vi "AddPotentialSweep.vi"(0 "deviceName":string, 1 "channel":u8, 2 "repeats":u16=1, 3 "quietTime":sgl, 4 "quietTimeSamplingInterval":sgl=1.0, 5 "startingPot":sgl, 6 "isStartVoltageVsOCP":bool, 7 "error in (no error)":errorcluster, 8 "endingPot":sgl, 9 "isEndVoltageVsOCP":bool, 10 "scanRate":sgl, 11 "samplingInterval":sgl, 12 "approxMaxCurrent":sgl=inf, 13 "isAutoRange":bool=TRUE, 14 "maxAbsoluteCurrent":sgl=inf, 15 "minAbsoluteCurrent":sgl, 16 "alphaFactor":sgl=75.0) -> (27 "error out":errorcluster)   [LabVIEW 2018]
doc: "EXPORT void AisAddPotentialSweep(const char* deviceName, uint8_t channel, uint16_t repeats, float quietTime, float quietTimeSamplingInterval, float startingPot, bool isStartVoltageVsOCP, float endingPot, bool isEndVoltageVsOCP, float scanRate, float samplingInterval, float approxMaxCurrent, bool isAutoRange, float maxAbsoluteCurrent, float minAbsoluteCurrent, float alphaFactor);"
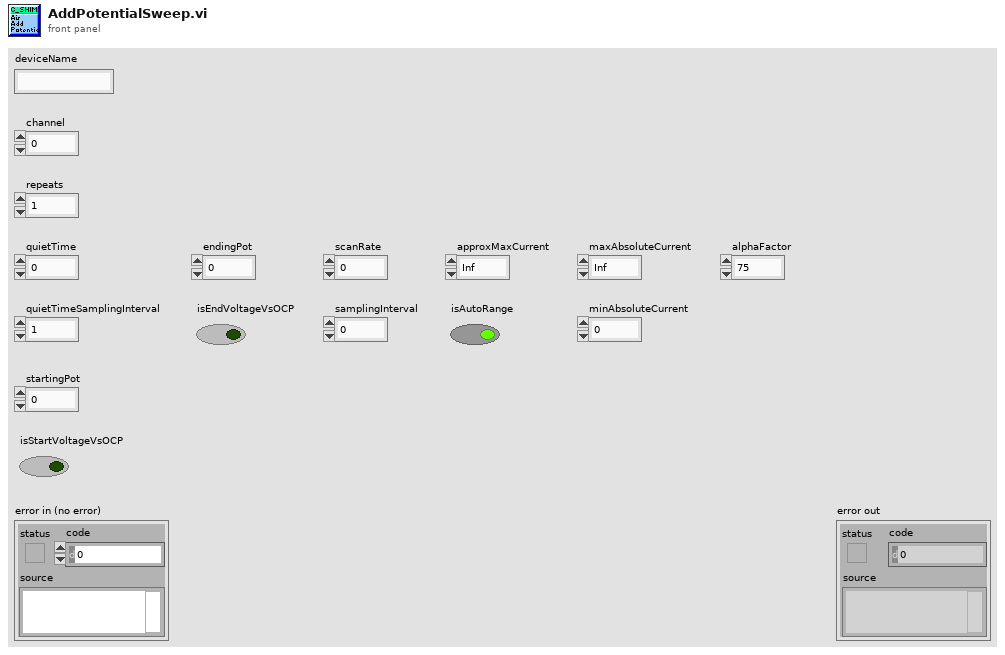
[diagram p1: front panel]
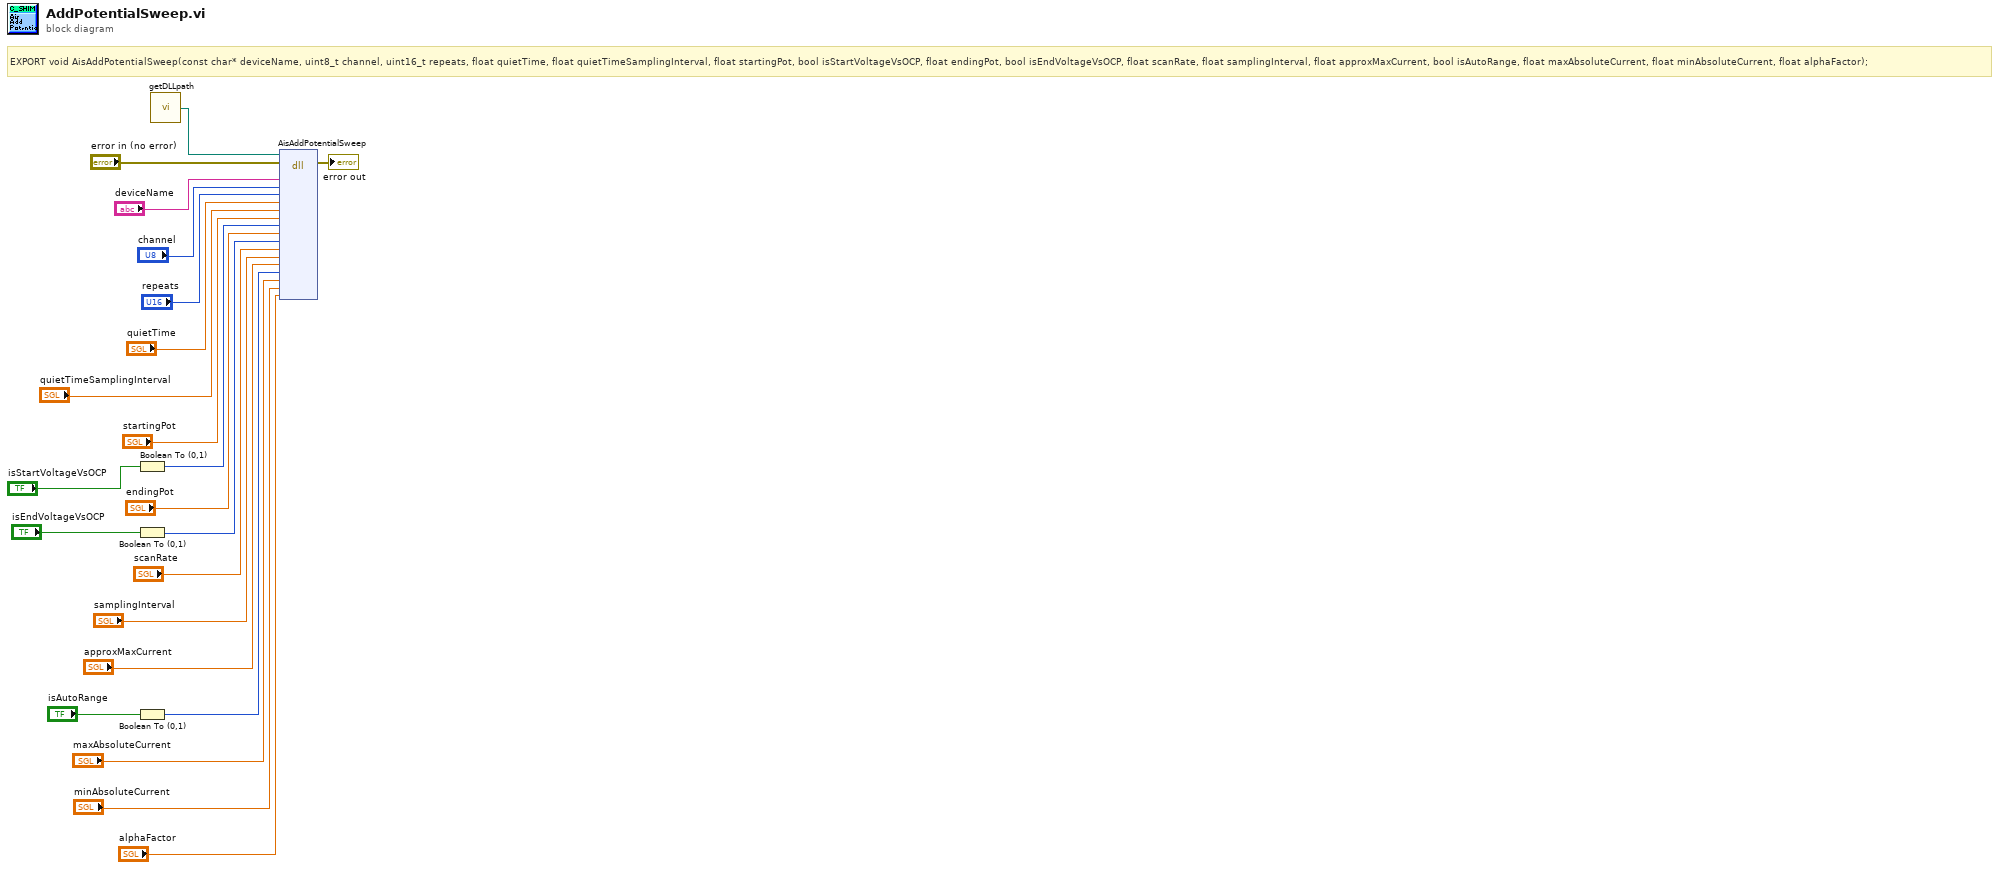
[diagram p0: block diagram]
diagram:
  # "EXPORT void AisAddPotentialSweep(const char* deviceName, uint8_t channel, uint16_t repeats, float quietTime, float quietTimeSamplingInterval, float startingPot, bool isStartVoltageVsOCP, float endingPot, bool isEndVoltageVsOCP, float scanRate, float samplingInterval, float approxMaxCurrent, bool isAutoRange, float maxAbsoluteCurrent, float minAbsoluteCurrent, float alphaFactor);"
  n1 = Boolean To (0,1)(Boolean="isStartVoltageVsOCP") -> (0, 1=w15:i16)
  n2 = Boolean To (0,1)(Boolean="isEndVoltageVsOCP") -> (0, 1=w12:i16)
  n3 = Boolean To (0,1)(Boolean="isAutoRange") -> (0, 1=w7:i16)
  n4 = call "getDLLpath.vi"() -> ("DLL_Path"=w1:path)
  n5 = dll-call lib="?" fn="AisAddPotentialSweep"(path in=w1, error in="error in (no error)", "deviceName"="deviceName", "channel"="channel", "repeats"="repeats", "quietTime"="quietTime", "quietTimeSamplingInterval"="quietTimeSamplingInterval", "startingPot"="startingPot", "isStartVoltageVsOCP"=w15, "endingPot"="endingPot", "isEndVoltageVsOCP"=w12, "scanRate"="scanRate", "samplingInterval"="samplingInterval", "approxMaxCurrent"="approxMaxCurrent", "isAutoRange"=w7, "maxAbsoluteCurrent"="maxAbsoluteCurrent", "minAbsoluteCurrent"="minAbsoluteCurrent", "alphaFactor"="alphaFactor") -> (error out=→"error out":errorcluster)  [unwired: 18 in, 1 out]
